vi "Test Assert Equal - deprecated.vi"(8 "error in (no error)":errorcluster) -> (0 "error out":errorcluster)   [LabVIEW 2013]
uses:
  classes/Assert/Assert.lvclass
  classes/Test/Test.lvclass
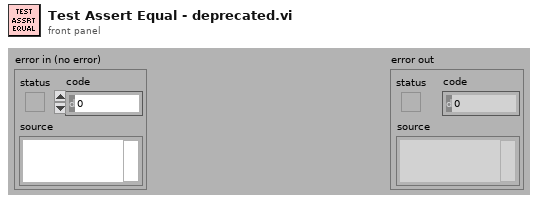
[diagram p1: front panel]
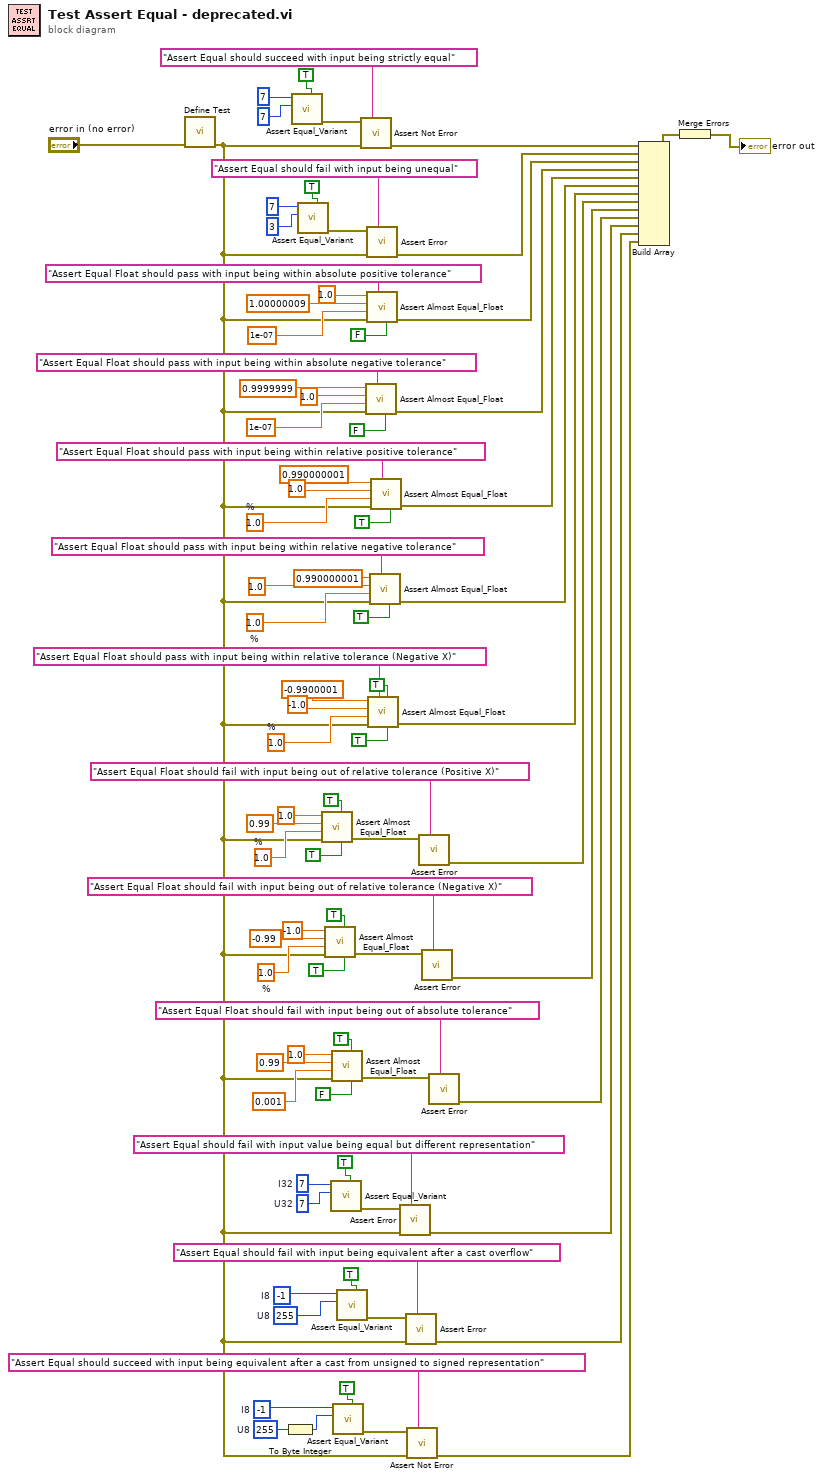
[diagram p0: block diagram]
diagram:
  w16 = u8 255  # U8
  w15 = i8 -1  # I8
  w17 = u8 255  # U8
  w18 = i8 -1  # I8
  w28 = u32 7  # U32
  w27 = 7  # I32
  w34 = 1.0  # %
  w40 = 1.0  # %
  w53 = 1.0  # %
  w60 = 1.0  # %
  w63 = 1.0  # %
  n1 = call "Define Test.vi"("error in (no error)"="error in (no error)") -> ("error out"=w11:errorcluster)  [unwired: 9 in, 1 out]
  n2 = To Byte Integer(number=w16) -> (8bit integer=w13:i8)
  n3 = call "Assert Equal_Variant.vi"("Assert Only? (F)"=TRUE, "Y"=7, "X"=7) -> ("error out"=w90:errorcluster)  [unwired: 8 in]
  n4 = call "Assert Equal_Variant.vi"("Assert Only? (F)"=TRUE, "Y"=3, "X"=7) -> ("error out"=w88:errorcluster)  [unwired: 8 in]
  n5 = call "Assert Almost Equal_Float.vi"("Use Percentage of X (F)"=TRUE, "Assert Only? (F)"=TRUE, "error in (no error)"=w11, "Tolerance"=w53, "Y"=0.99, "X"=1.0) -> ("error out"=w51:errorcluster)  [unwired: 4 in, 1 out]
  n6 = call "Assert Almost Equal_Float.vi"("Use Percentage of X (F)"=TRUE, "Assert Only? (F)"=TRUE, "error in (no error)"=w11, "Tolerance"=w34, "Y"=-0.99, "X"=-1.0) -> ("error out"=w36:errorcluster)  [unwired: 4 in, 1 out]
  n7 = call "Assert Equal_Variant.vi"("Assert Only? (F)"=TRUE, "Y"=w28, "X"=w27) -> ("error out"=w21:errorcluster)  [unwired: 8 in]
  n8 = call "Assert Almost Equal_Float.vi"("Use Percentage of X (F)"=FALSE, "Assert Only? (F)"=TRUE, "error in (no error)"=w11, "Tolerance"=0.001, "Y"=0.99, "X"=1.0) -> ("error out"=w49:errorcluster)  [unwired: 4 in, 1 out]
  n9 = call "Assert Equal_Variant.vi"("Assert Only? (F)"=TRUE, "Y"=w13, "X"=w15) -> ("error out"=w12:errorcluster)  [unwired: 8 in]
  n10 = call "Assert Equal_Variant.vi"("Assert Only? (F)"=TRUE, "Y"=w17, "X"=w18) -> ("error out"=w23:errorcluster)  [unwired: 8 in]
  n11 = call "Assert Not Error.vi"("Label"="Assert Equal should succeed with input being strictly equal", "error in (no error)"=w11, "Not Error?"=w90) -> ("error out"=w78:errorcluster)  [unwired: 7 in, 1 out]
  n12 = call "Assert Almost Equal_Float.vi"("Use Percentage of X (F)"=FALSE, "Label"="Assert Equal Float should pass with input being within absolute negative tolerance", "error in (no error)"=w11, "Tolerance"=1e-07, "Y"=1.0, "X"=0.9999999) -> ("error out"=w66:errorcluster)  [unwired: 4 in, 1 out]
  n13 = call "Assert Error.vi"("Label"="Assert Equal should fail with input being unequal", "error in (no error)"=w11, "Error?"=w88) -> ("error out"=w77:errorcluster)  [unwired: 7 in, 1 out]
  n14 = call "Assert Almost Equal_Float.vi"("Use Percentage of X (F)"=FALSE, "Label"="Assert Equal Float should pass with input being within absolute positive tolerance", "error in (no error)"=w11, "Tolerance"=1e-07, "Y"=1.00000009, "X"=1.0) -> ("error out"=w74:errorcluster)  [unwired: 4 in, 1 out]
  n15 = call "Assert Almost Equal_Float.vi"("Use Percentage of X (F)"=TRUE, "Assert Only? (F)"=TRUE, "Label"="Assert Equal Float should pass with input being within relative tolerance (Negative X)", "error in (no error)"=w11, "Tolerance"=w40, "Y"=-1.0, "X"=-0.9900001) -> ("error out"=w37:errorcluster)  [unwired: 3 in, 1 out]
  n16 = call "Assert Almost Equal_Float.vi"("Use Percentage of X (F)"=TRUE, "Label"="Assert Equal Float should pass with input being within relative negative tolerance", "error in (no error)"=w11, "Tolerance"=w60, "Y"=1.0, "X"=0.990000001) -> ("error out"=w58:errorcluster)  [unwired: 4 in, 1 out]
  n17 = call "Assert Almost Equal_Float.vi"("Use Percentage of X (F)"=TRUE, "Label"="Assert Equal Float should pass with input being within relative positive tolerance", "error in (no error)"=w11, "Tolerance"=w63, "Y"=1.0, "X"=0.990000001) -> ("error out"=w59:errorcluster)  [unwired: 4 in, 1 out]
  n18 = call "Assert Error.vi"("Label"="Assert Equal should fail with input value being equal but different representation", "error in (no error)"=w11, "Error?"=w21) -> ("error out"=w20:errorcluster)  [unwired: 7 in, 1 out]
  n19 = call "Assert Error.vi"("Label"="Assert Equal should fail with input being equivalent after a cast overflow", "error in (no error)"=w11, "Error?"=w23) -> ("error out"=w22:errorcluster)  [unwired: 7 in, 1 out]
  n20 = call "Assert Not Error.vi"("Label"="Assert Equal should succeed with input being equivalent after a cast from unsigned to signed representation", "error in (no error)"=w11, "Not Error?"=w12) -> ("error out"=w9:errorcluster)  [unwired: 7 in, 1 out]
  n21 = call "Assert Error.vi"("Label"="Assert Equal Float should fail with input being out of relative tolerance (Positive X)", "Error?"=w51) -> ("error out"=w50:errorcluster)  [unwired: 8 in, 1 out]
  n22 = call "Assert Error.vi"("Label"="Assert Equal Float should fail with input being out of relative tolerance (Negative X)", "Error?"=w36) -> ("error out"=w29:errorcluster)  [unwired: 8 in, 1 out]
  n23 = call "Assert Error.vi"("Label"="Assert Equal Float should fail with input being out of absolute tolerance", "Error?"=w49) -> ("error out"=w42:errorcluster)  [unwired: 8 in, 1 out]
  n24 = Build Array(w78, w77, w74, w66, w59, w58, w37, w50, w29, w42, w20, w22, w9) -> (w76:errorcluster[])
  n25 = Merge Errors(w76) -> (→"error out":errorcluster)
